vi "Pulse line.vi"(8 "error in (no error)":errorcluster, 10 "Line number":u8, 11 "TTL in":refnum<class "TTL.lvclass">) -> (0 "error out":errorcluster, 3 "TTL out":refnum<class "TTL.lvclass">)   [LabVIEW 2014, in "TTL.lvclass"]
doc: "Pulses a TTL line. The line is set to \"ON\" for the duration of the \"pulse duration\" setting, followed by an \"OFF\" period, also governed by the \"pulse duration\" setting.\n(So, the total pulse takes 2 * pulse duration)."
uses:
  TTL.lvclass
  TTL.lvclass/TTL.ctl
  cosylib/COSYLib.lvlib
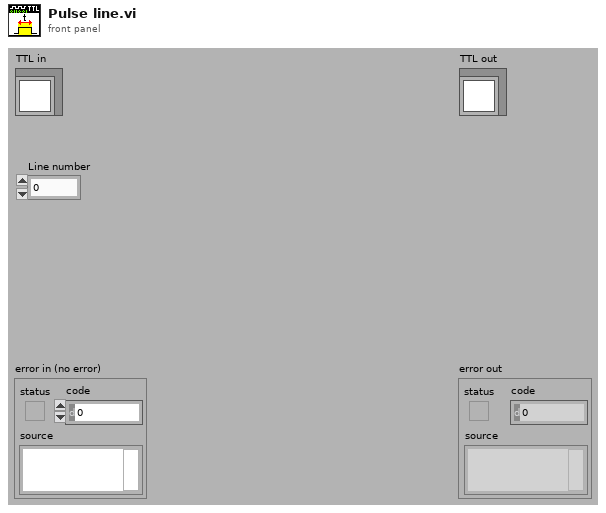
[diagram p1: front panel]
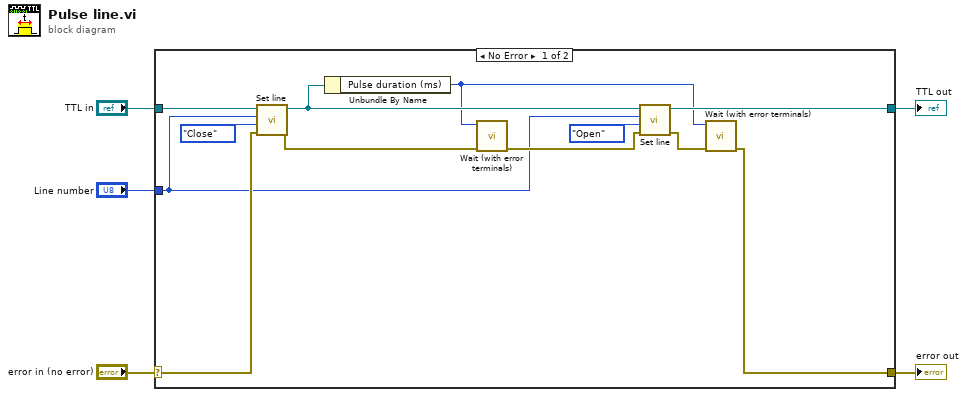
[diagram p0: block diagram]
diagram:
  n1 = case shown="No Error" "error in (no error)" {
    selector: "error in (no error)" -> [w15 w19]
    tunnel: [w7 w19] -> w4
    tunnel: [w13 w18] -> w2
    tunnel: "TTL in" -> [w12 w18]
    tunnel: "Line number" -> [w14 _]
    frame No Error {
      n2 = call "Set line.vi"("error in (no error)"=w15, "Action"=enum16{"Open", "Close", "Toggle"}."Close", "Line number"=w14, "TTL in"=w12) -> ("error out"=w16:errorcluster, "TTL out"=w11:refnum<class "TTL.lvclass">)  [unwired: 6 in]
      n3 = Unbundle By Name(w11) -> ("Pulse duration (ms)"=w6:u32)
      n4 = call "Wait (with error terminals).vi"("error in (no error)"=w16, "milliseconds to wait"=w6) -> ("error out"=w17:errorcluster)  [unwired: 8 in, 1 out]
      n5 = call "Set line.vi"("error in (no error)"=w17, "Action"=enum16{"Open", "Close", "Toggle"}."Open", "Line number"=w14, "TTL in"=w11) -> ("error out"=w8:errorcluster, "TTL out"=w13:refnum<class "TTL.lvclass">)  [unwired: 6 in]
      n6 = call "Wait (with error terminals).vi"("error in (no error)"=w8, "milliseconds to wait"=w6) -> ("error out"=w7:errorcluster)  [unwired: 8 in, 1 out]
    }
    frame Error {
    }
  }
  "error out" <- w4
  "TTL out" <- w2
